vi "Get Ingredients.vi"(8 "error in (no error)":errorcluster, 11 "Plastic Parts in":refnum<class "Plastic Parts.lvclass">) -> (0 "error out":errorcluster, 2 "Ingredients":T1[](array[typedef]), 3 "Plastic Parts out":refnum<class "Plastic Parts.lvclass">)   [LabVIEW 2020, in "Plastic Parts.lvclass"]
uses:
  Plastic Parts.lvclass
  Item/Ingredient.ctl
  Item/Item.lvclass
  Plastic/Plastic.lvclass
  C:/dev/LabVIEW/Good Company Calc/Item/Item.lvclass
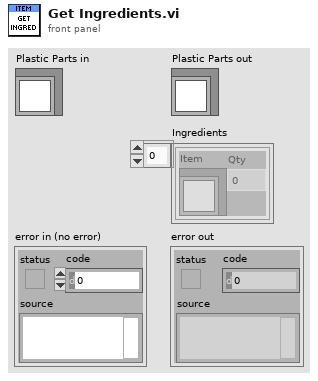
[diagram p1: front panel]
types:
  T1 = typedef "Item.lvclass/Ingredient.ctl" = cluster{"Item":refnum<class "Item.lvclass">, "Qty":dbl}
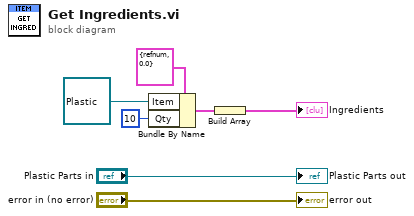
[diagram p0: block diagram]
diagram:
  n1 = Bundle By Name(cluster=T1 {"Item"=refnum, "Qty"=0.0} ("input cluster"), "Item"=refnum<class "Plastic.lvclass"> refnum ("Plastic.lvclass"), "Qty"=10) -> (w2:T1)
  n2 = Build Array(w2) -> (→"Ingredients":T1[])
  "error out" <- "error in (no error)"
  "Plastic Parts out" <- "Plastic Parts in"
